vi "rad_Check Image RT-INI For AutoRun.vi"(5 "password":string, 8 "error in (no error)":errorcluster, 9 "target settings":T1={"Hostname"="", "Serial number"="", "Product name"="", "Product code"=0, "System status"="", "Credential type"=enum."None/Unlocked", "User added?"=FALSE, "Primary NIC"={"MAC address"="", "IP Address Request Mode"=2, "IP address"="", "Subnet mask"="", "Gateway"="", "DNS server"=""}} {"Primary NIC"."IP Address Request Mode" items=["Static"=1, "DHCP/Link-Local"=2, "Link-Local Only"=4, "DHCP Only"=8]}, 11 "temp folder":path) -> (0 "error out":errorcluster, 2 "Run at Startup?":bool, 3 "temp folder out":path)   [LabVIEW 2020]
uses:
  <vilib>/Utility/config.llb/NI_LVConfig.lvlib
  <vilib>/Utility/config.llb/Read Key (Boolean).vi
  <resource>/objmgr/nicriosae.rc
  <resource>/objmgr/nisysapi.rc
  <vilib>/nisyscfg/nisyscfg.lvlib
  <vilib>/nisyscfg/Close (System).vi
  <vilib>/nisyscfg/Close (Hardware).vi
  Targets/TypeDefs/rad_Target Information.ctl
  Targets/TypeDefs/rad_Target Network Settings.ctl
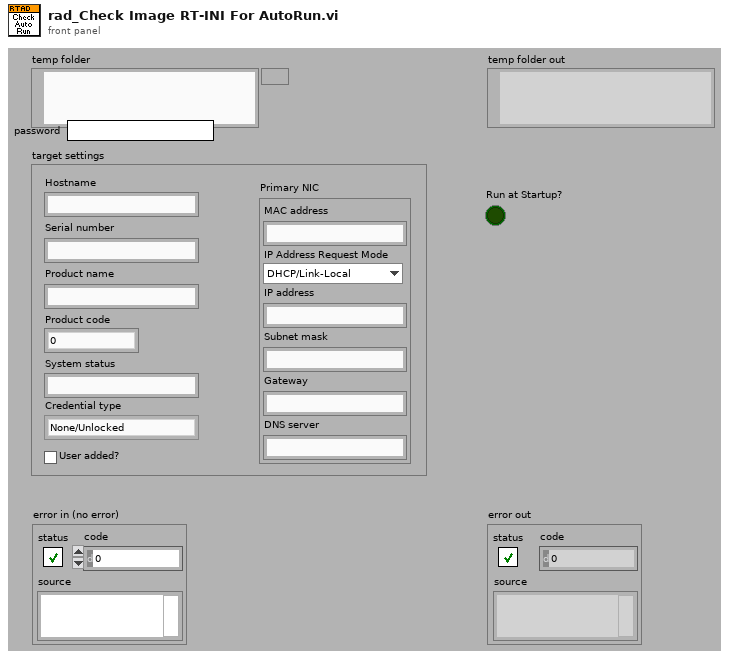
[diagram p1: front panel]
types:
  T1 = typedef "rad_Target Information.ctl" = cluster{"Hostname":string, "Serial number":string, "Product name":string, "Product code":i32, "System status":string, "Credential type":enum16{"None/Unlocked", "FTP Password", "NIAuth Credentials"}, "User added?":bool, "Primary NIC":T2}
  T2 = typedef "rad_Target Network Settings.ctl" = cluster{"MAC address":string, "IP Address Request Mode":i32, "IP address":string, "Subnet mask":string, "Gateway":string, "DNS server":string}
  T3 = enum16{"None/Unlocked", "FTP Password", "NIAuth Credentials"}
  T4 = typedef "NI_LVConfig.lvlib/Config Data RefNum.ctl" = refnum<k1>
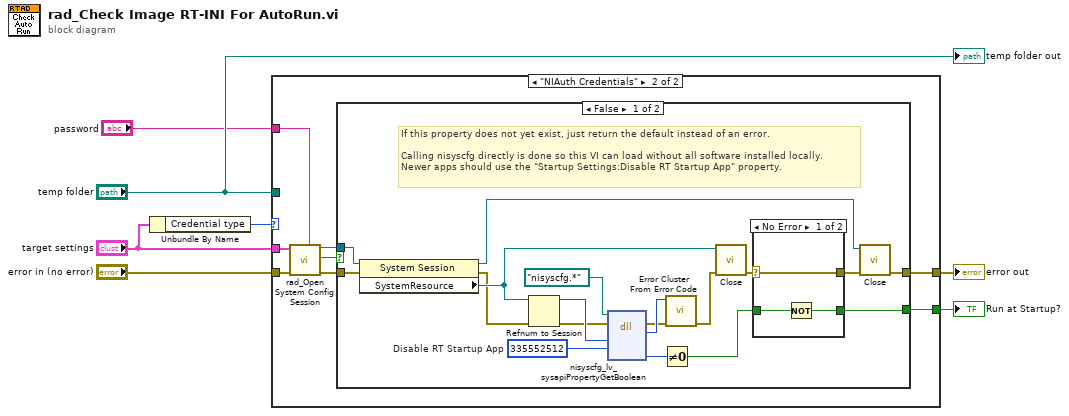
[diagram p0: block diagram]
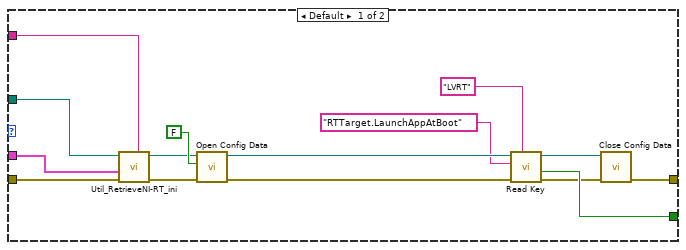
[diagram p2: hidden frame]
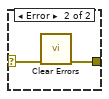
[diagram p3: hidden frame]
diagram:
  n1 = Unbundle By Name("target settings") -> ("Credential type"=w4:T3)
  n2 = case shown="\"NIAuth Credentials\"" w4 {
    tunnel: [w19 w25] -> w7
    tunnel: [w16 w24] -> w6
    tunnel: "temp folder" -> [w13 _]
    tunnel: "target settings" -> [w9 w30]
    tunnel: "error in (no error)" -> [w11 w29]
    tunnel: "password" -> [w8 w23]
    frame Default {
      n3 = call "Util_RetrieveNI-RT_ini.vi"("password"=w8, "error in"=w11, "Target settings"=w9, "temp folder"=w13) -> ("error out"=w10:errorcluster, "Ini File Path"=w12:path)  [unwired: 6 in]
      n4 = call <vilib>:"Open Config Data.vi"("error in (no error)"=w10, "create file if necessary (T)"=FALSE, "configuration file path"=w12) -> ("error out"=w20:errorcluster, "refnum"=w21:T4)  [unwired: 6 in, 1 out]
      n5 = call-poly <vilib>:"Read Key.vi"("section"="LVRT", "error in (no error)"=w20, "key"="RTTarget.LaunchAppAtBoot", "refnum"=w21) -> ("error out"=w15:errorcluster, "value"=w19:bool, "refnum out"=w14:T4)  [unwired: 4 in, 1 out]
      n6 = call <vilib>:"Close Config Data.vi"("error in (no error)"=w15, "refnum"=w14) -> ("error out"=w16:errorcluster)  [unwired: 8 in, 1 out]
    }
    frame "NIAuth Credentials" {
      n7 = call "rad_Open System Config Session.vi"("Password"=w23, "error in (no error)"=w29, "Target settings"=w30) -> ("error out"=w26:errorcluster, "Cancelled"=w27:bool, "Session out"=w28:refnum<k21>)  [unwired: 5 in, 1 out]
      n8 = case shown="False" w27 {
        tunnel: w28 -> [w48 _]
        tunnel: w26 -> [w47 w54]
        tunnel: [w45 w54] -> w24
        tunnel: [w42 _] -> w25
        frame False {
          w40 = u32 335552512  # Disable RT Startup App
          # "If this property does not yet exist, just return the default instead of an error.\n\nCalling nisyscfg directly is done so this VI can load without all software installed locally.\nNewer apps should use the \"Startup Settings:Disable RT Startup App\" property."
          n9 = property class="System Session"(reference=w48, error in=w47) -> (reference out=w46:refnum<k21>, error out=w34:errorcluster, "SystemResource"=w35:refnum<k20>)
          n10 = Refnum to Session(4:w34, 7:w35) -> (0:w36:errorcluster, 3:w41:u64)
          n11 = dll-call lib="nisyscfg.dll" fn="nisyscfg_lv_sysapiPropertyGetBoolean"(path in=path "nisyscfg.*", error in=w36, "resource"=w41, "attribute"=w40) -> (error out=w37:errorcluster, "status"=w39:i32, "value"=w32:u8)  [unwired: 4 in, 1 out]
          n12 = Not Equal To 0?(x=w32) -> (x != 0?=w31:bool)
          n13 = call <vilib>:"Error Cluster From Error Code.vi"("error in (no error)"=w37, "error code (0)"=w39) -> ("error out"=w33:errorcluster)  [unwired: 2 in, 5 out]
          n14 = call-poly <vilib>:"Close.vi"("error in (no error)"=w33, "Resource in"=w35) -> ("error out"=w44:errorcluster)  [unwired: 9 in]
          n15 = case shown="No Error" w44 {
            selector: w44 -> [w51 w53]
            tunnel: [w51 w52] -> w43
            tunnel: [w50 _] -> w42
            tunnel: w31 -> [w49 _]
            frame No Error {
              n16 = Not(x=w49) -> (.not. x?=w50:bool)
            }
            frame Error {
              n17 = call <vilib>:"Clear Errors.vi"("error in (no error)"=w53) -> ("error out"=w52:errorcluster)  [unwired: 5 in, 1 out]
            }
          }
          n18 = call-poly <vilib>:"Close.vi"("error in (no error)"=w43, "Session in"=w46) -> ("error out"=w45:errorcluster)  [unwired: 9 in]
        }
        frame True {
        }
      }
    }
  }
  "Run at Startup?" <- w7
  "error out" <- w6
  "temp folder out" <- "temp folder"
